vi "BRig_dataExp_ClosedLoop_LaserHold_l2.vi"() -> (2 "output_CloseLoop_LaserHold_l2":i32)   [LabVIEW 2014]
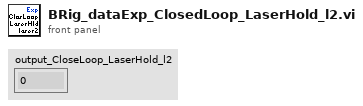
[diagram p1: front panel]
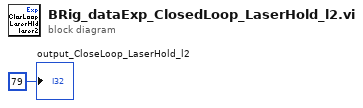
[diagram p0: block diagram]
diagram:
  "output_CloseLoop_LaserHold_l2" <- 79 ("output_iBlock")
